vi "Read Attributes.vi"(11 "Activate or Blackstart Msg":refnum<class "Activate or Blackstart Msg.lvclass">) -> (2 "Payload":cluster{"Activate or Blackstart":T1})   [LabVIEW 2018, in "Commissioning Actor.lvlib" / "Activate or Blackstart Msg.lvclass"]
uses:
  Activate or Blackstart Msg.lvclass
  Commissioning/Controls/Activate or Blackstart Selector.ctl
  Activate or Blackstart Msg.lvclass/Activate or Blackstart Msg.ctl
  Commissioning/Commissioning.lvclass
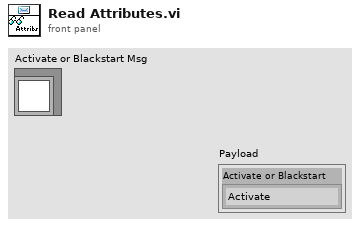
[diagram p1: front panel]
types:
  T1 = typedef "Commissioning Actor.lvlib/Commissioning.lvclass/Activate or Blackstart Selector.ctl" = enum16{"Activate", "Blackstart"}
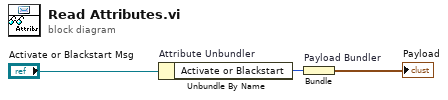
[diagram p0: block diagram]
diagram:
  n1 = Unbundle By Name "Attribute Unbundler"("Activate or Blackstart Msg") -> ("Activate or Blackstart"=w1:T1)
  n2 = Bundle "Payload Bundler"("Activate or Blackstart"=w1) -> (→"Payload":cluster{"Activate or Blackstart":T1})  [unwired: 1 in]
